vi "StateTransitionEdge_Create.vi"(0 "reference":refnum<class "StateTransitionEdge.lvclass">, 5 "error in (no error)":errorcluster, 6 "GoopReferenceIn":T1) -> (14 "reference out":refnum<class "StateTransitionEdge.lvclass">, 16 "# of objects":i32, 19 "error out":errorcluster)   [LabVIEW 2012, in "StateTransitionEdge.lvclass"]
doc: "Creates and initializes a new StateTransitionEdge object.\n\nThis object should be destroyed using a StateTransitionEdge destructor VI or a virtual base class destructor VI.\n\n[GOOP 2.1]"
uses:
  <resource>/Framework/Providers/Open_GDS/UML/StateTransitionEdge_class/StateTransitionEdge.lvclass
  <resource>/Framework/Providers/Open_GDS/UML/AbstractEdge_class/ObjectReference.ctl
  <resource>/Framework/Providers/Open_GDS/UML/ArrowHead_class/ArrowHeadType.ctl
  <resource>/Framework/Providers/Open_GDS/UML/BentStyle_class/BentStyleType.ctl
  <resource>/Framework/Providers/Open_GDS/UML/LineStyle_class/LineStyleType.ctl
  <resource>/Framework/Providers/Open_GDS/UML/ClassRelationshipEdge_class/ClassRelationshipEdge.lvclass
  <resource>/Framework/Providers/Open_GDS/UML/LineStyle_class/LineStyle.lvclass
  <resource>/Framework/Providers/Open_GDS/UML/ArrowHead_class/ArrowHead.lvclass
  <resource>/Framework/Providers/Open_GDS/UML/BentStyle_class/BentStyle.lvclass
  <resource>/Framework/Providers/Open_GDS/UML/AbstractEdge_class/AbstractEdge.lvclass
panel:
  # "The input reference should only\nbe wired when this method is called\nby a sub class constructor."
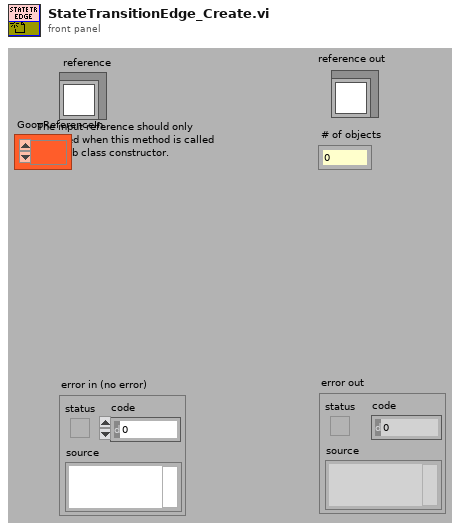
[diagram p1: front panel]
types:
  T1 = typedef "AbstractEdge.lvclass/ObjectReference.ctl" = refnum<k1>
  T2 = typedef "LineStyle.lvclass/LineStyleType.ctl" = enum16{"SOLID", "DOTTED"}
  T3 = typedef "BentStyle.lvclass/BentStyleType.ctl" = enum16{"STRAIGHT", "HV", "VH", "HVH", "VHV", "ARC"}
  T4 = typedef "ArrowHead.lvclass/ArrowHeadType.ctl" = enum16{"NONE", "TRIANGLE", "BLACK_TRIANGLE", "V", "HALF_V", "DIAMOND", "BLACK_DIAMOND"}
  T5 = typedef "StateTransitionEdge.lvclass/ObjectAttributes.ctl" = cluster{"Base class":T6, "angle":dbl}
  T6 = typedef "ClassRelationshipEdge.lvclass/ObjectAttributes.ctl" = cluster{"Base class":T7, "bentStyleRef":refnum<class "BentStyle.lvclass">, "startConnectionOffset":cluster{"x":i32, "y":i32}, "endConnectionOffset":cluster{"x":i32, "y":i32}, "MidLineOffset":cluster{"x":i32, "y":i32}, "DepClass":T11}
  T7 = typedef "SegmentedLineEdge.lvclass/ObjectAttributes.ctl" = cluster{"Base class":T8, "lineStyle":refnum<class "LineStyle.lvclass">, "startArrowHead":refnum<class "ArrowHead.lvclass">, "endArrowHead":refnum<class "ArrowHead.lvclass">, "startLabel":string, "midLabel":string, "endLabel":string, "MidLabelOffset":T10, "SplitWire":bool}
  T8 = typedef "GeneralPathEdge.lvclass/ObjectAttributes.ctl" = cluster{"Base class":T9}
  T9 = typedef "AbstractEdge.lvclass/ObjectAttributes.ctl" = cluster{"start":refnum<class "AbstractNode.lvclass">, "end":refnum<class "AbstractNode.lvclass">}
  T10 = typedef "Point Point2D.ctl" = cluster{"x":dbl, "y":dbl}
  T11 = typedef "ReversedEngineering_ViDependencyDetailsType.ctl" = cluster{"ThisVIs/Ctls":path[], "Dependent_VIs/Ctls":path[]}
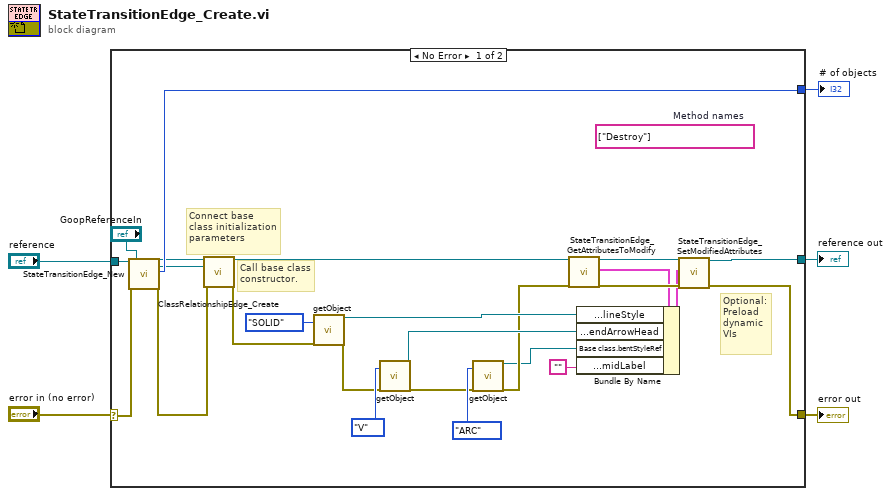
[diagram p0: block diagram]
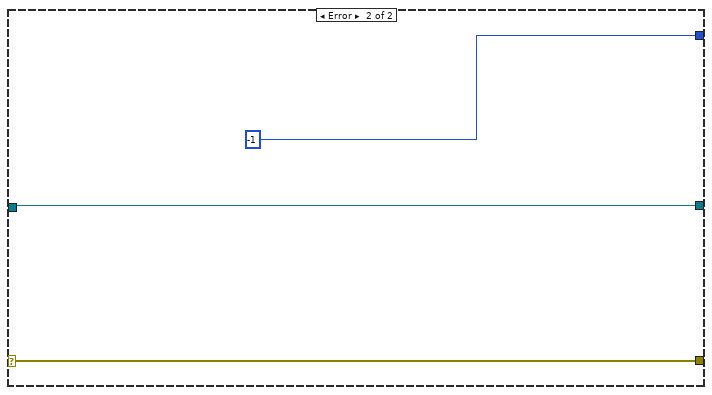
[diagram p2: hidden frame]
diagram:
  n1 = case shown="No Error" "error in (no error)" {
    selector: "error in (no error)" -> [w30 w32]
    tunnel: [w20 w31] -> w5
    tunnel: [w19 w32] -> w4
    tunnel: [w29 -1 ("Nr of open handles")] -> w3
    tunnel: "reference" -> [w28 w31]
    frame No Error {
      (unwired) string[] ["Destroy"]  # Method names
      # "Optional:\nPreload\ndynamic\nVIs"
      # "Connect base\nclass initialization\nparameters"
      # "Call base class\nconstructor."
      n2 = call <resource>:"StateTransitionEdge_New.vi"("reference in"=w28, "error in (no error)"=w30, "GoopReferenceIn"="GoopReferenceIn") -> ("GoopReferenceOut"=w7:T1, "reference out"=w25:refnum<class "StateTransitionEdge.lvclass">, "# of objects"=w29:i32, "error out"=w27:errorcluster)  [unwired: 2 in, 11 out]
      n3 = call <resource>:"ClassRelationshipEdge_Create.vi"("reference"=w25, "error in (no error)"=w27, "GoopReferenceIn"=w7) -> ("reference out"=w24:refnum<class "StateTransitionEdge.lvclass">, "error out"=w16:errorcluster)  [unwired: 15 out]
      n4 = call <resource>:"getObject.vi"("lineStyle"=LineStyleType."SOLID", "error in (no error)"=w16) -> ("reference out"=w18:refnum<class "LineStyle.lvclass">, "error out"=w13:errorcluster)  [unwired: 16 out]
      n5 = call <resource>:"getObject.vi"("arrowHead"=ArrowHeadType."V", "error in (no error)"=w13) -> ("reference out"=w14:refnum<class "ArrowHead.lvclass">, "error out"=w11:errorcluster)  [unwired: 16 out]
      n6 = call <resource>:"getObject.vi"("bentStyle"=BentStyleType."ARC", "error in (no error)"=w11) -> ("reference out"=w9:refnum<class "BentStyle.lvclass">, "error out"=w10:errorcluster)  [unwired: 16 out]
      n7 = call <resource>:"StateTransitionEdge_GetAttributesToModify.vi"("reference in"=w24, "error in (no error)"=w10) -> ("reference out"=w23:refnum<class "StateTransitionEdge.lvclass">, "Attributes"=w22:T5, "error out"=w26:errorcluster)  [unwired: 1 in, 14 out]
      n8 = Bundle By Name(cluster=w22, "Base class.Base class.lineStyle"=w18, "Base class.Base class.endArrowHead"=w14, "Base class.bentStyleRef"=w9, "Base class.Base class.midLabel"="") -> (w21:T5)
      n9 = call <resource>:"StateTransitionEdge_SetModifiedAttributes.vi"("reference in"=w23, "Attributes"=w21, "error in (no error)"=w26) -> ("reference out"=w20:refnum<class "StateTransitionEdge.lvclass">, "error out"=w19:errorcluster)  [unwired: 3 in, 12 out]
    }
    frame Error {
    }
  }
  "error out" <- w4
  "reference out" <- w5
  "# of objects" <- w3
